vi "GrabImageDisplay.vi"(0 "nPixelFormat":i32, 1 "pInputBuffer":u8[](array[numeric]), 5 "nWidth":u32, 7 "nHeight":u32, 9 "Image Src":T1, 11 "error in (no error)":errorcluster) -> (4 "Image out":T1, 15 "error out":errorcluster)   [LabVIEW 2016, in "GxLVLib.lvlib"]
uses:
  GxLVLib.lvlib
  <vilib>/vision/Image Controls.llb/IMAQ Image.ctl
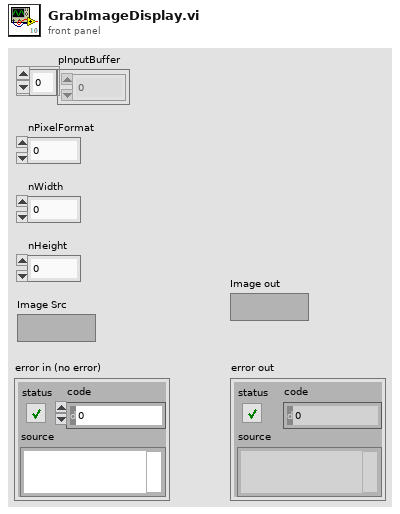
[diagram p1: front panel]
types:
  T1 = typedef "IMAQ Image.ctl" = refnum<image>
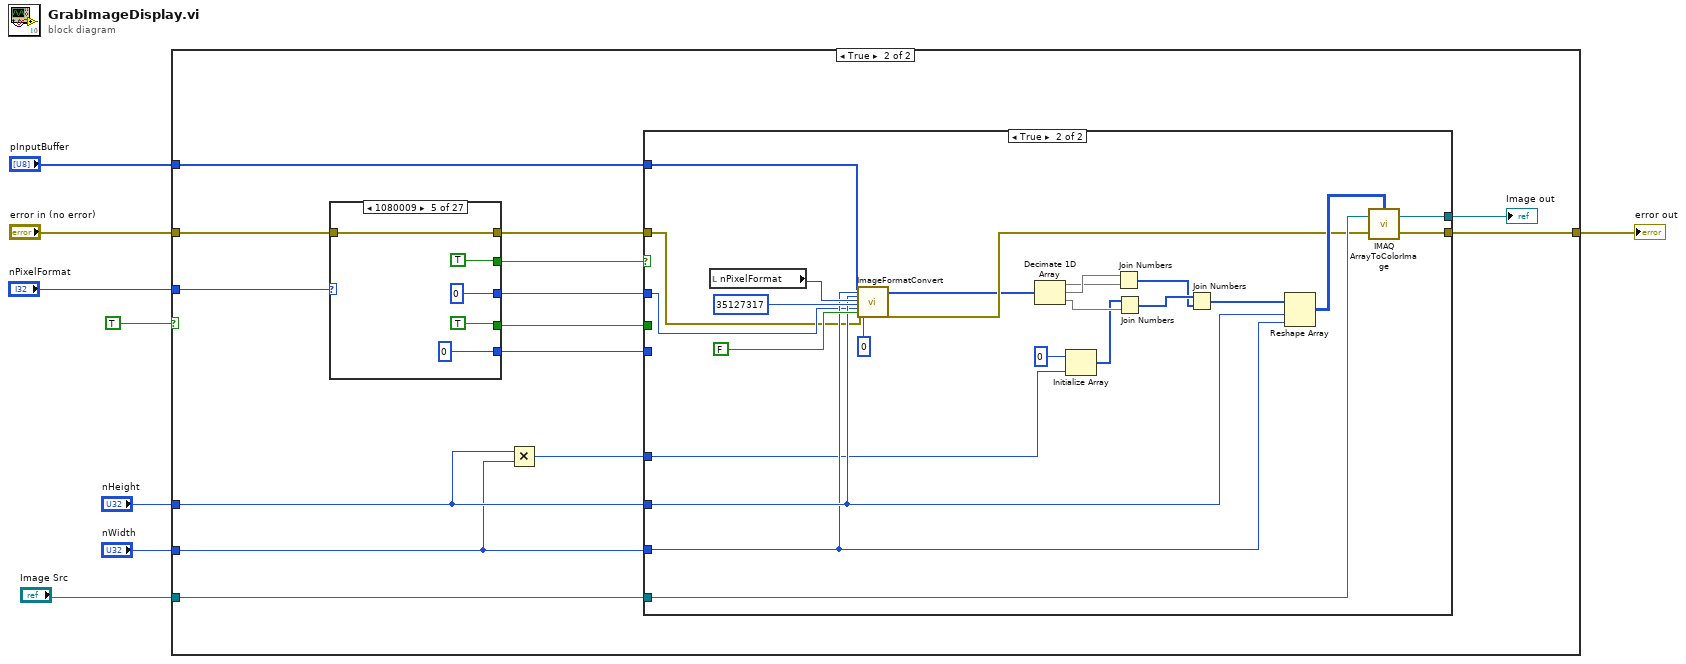
[diagram p0: block diagram]
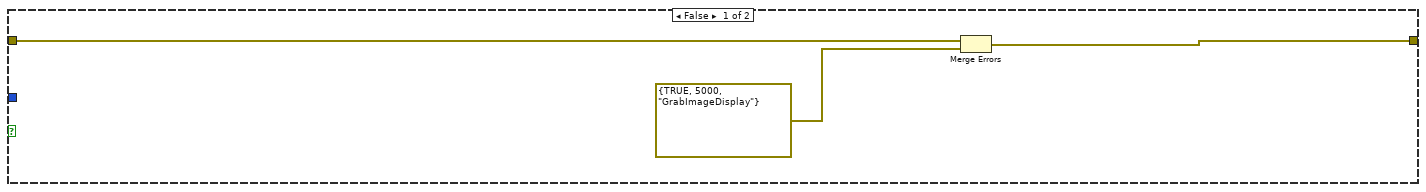
[diagram p2: hidden frame]
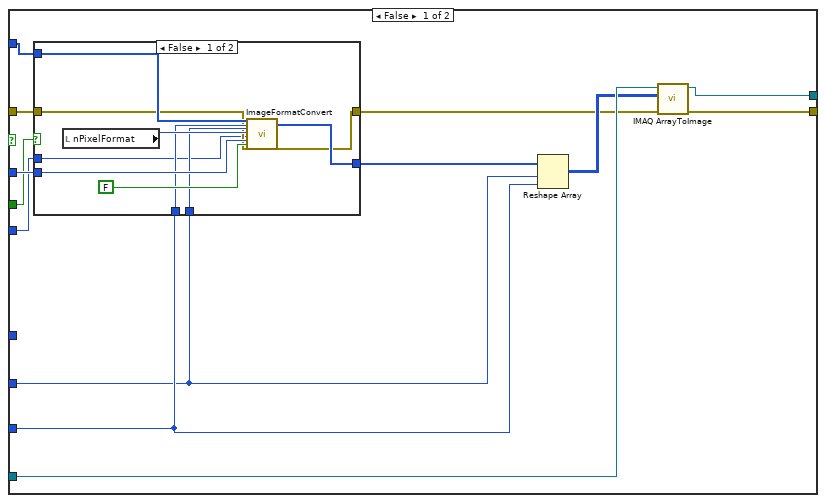
[diagram p3: hidden frame]
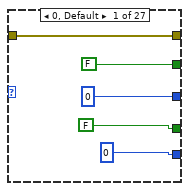
[diagram p5: hidden frame]
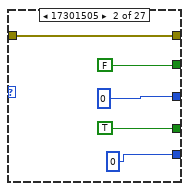
[diagram p6: hidden frame]
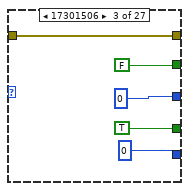
[diagram p7: hidden frame]
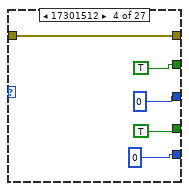
[diagram p8: hidden frame]
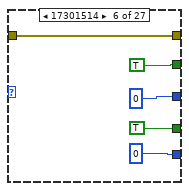
[diagram p9: hidden frame]
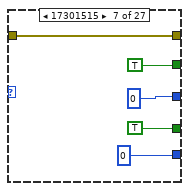
[diagram p10: hidden frame]
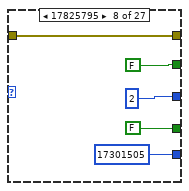
[diagram p11: hidden frame]
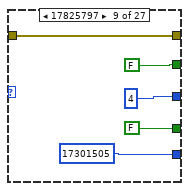
[diagram p12: hidden frame]
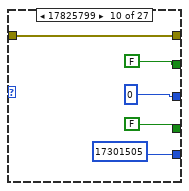
[diagram p13: hidden frame]
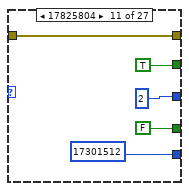
[diagram p14: hidden frame]
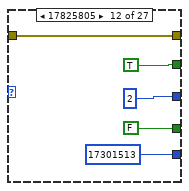
[diagram p15: hidden frame]
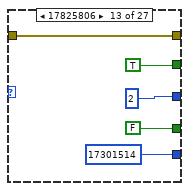
[diagram p16: hidden frame]
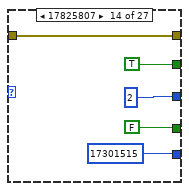
[diagram p17: hidden frame]
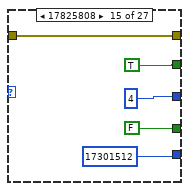
[diagram p18: hidden frame]
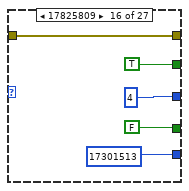
[diagram p19: hidden frame]
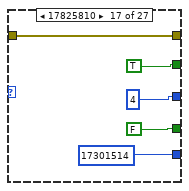
[diagram p20: hidden frame]
diagram:
  n1 = case shown="True" TRUE ("Boolean") {
    tunnel: "error in (no error)" -> [w11 w17]
    tunnel: [w9 w20] -> w7
    tunnel: "Image Src" -> [_ w21]
    tunnel: "nPixelFormat" -> [_ w16]
    tunnel: "nHeight" -> [_ w15]
    tunnel: "nWidth" -> [_ w14]
    tunnel: "pInputBuffer" -> [_ w13]
    frame False {
      n2 = Merge Errors(w11, errorcluster {TRUE, 5000, "GrabImageDisplay"}) -> (w9:errorcluster)
    }
    frame True {
      n3 = case shown="1080009" w16 {
        tunnel: [0 0 0 0 0 0 0 2 4 0 2 2 2 2 4 4 4 4 0 0 0 0 0 0 2 4 0] -> w24
        tunnel: [FALSE FALSE FALSE TRUE TRUE TRUE TRUE FALSE FALSE FALSE TRUE TRUE TRUE TRUE TRUE TRUE TRUE TRUE FALSE TRUE TRUE TRUE TRUE TRUE TRUE TRUE TRUE] -> w25
        tunnel: [FALSE TRUE TRUE TRUE TRUE TRUE TRUE FALSE FALSE FALSE FALSE FALSE FALSE FALSE FALSE FALSE FALSE FALSE FALSE FALSE FALSE FALSE FALSE FALSE FALSE FALSE FALSE] -> w23
        tunnel: w17 -> [w76 w81 w89 w94 w99 w104 w109 w114 w119 w124 w129 w134 w139 w144 w149 w154 w159 w164 w169 w174 w179 w184 w189 w194 w199 w204 w209]
        tunnel: [w76 w81 w89 w94 w99 w104 w109 w114 w119 w124 w129 w134 w139 w144 w149 w154 w159 w164 w169 w174 w179 w184 w189 w194 w199 w204 w209] -> w22
        tunnel: [0 ("DstPixelFormat") 0 ("DstPixelFormat") 0 ("DstPixelFormat") 0 ("DstPixelFormat") 0 ("DstPixelFormat") 0 ("DstPixelFormat") 0 ("DstPixelFormat") 17301505 ("DstPixelFormat") 17301505 ("DstPixelFormat") 17301505 ("DstPixelFormat") 17301512 ("DstPixelFormat") 17301513 ("DstPixelFormat") 17301514 ("DstPixelFormat") 17301515 ("DstPixelFormat") 17301512 ("DstPixelFormat") 17301513 ("DstPixelFormat") 17301514 ("DstPixelFormat") 17301515 ("DstPixelFormat") 17301505 ("DstPixelFormat") 17301512 ("DstPixelFormat") 17301513 ("DstPixelFormat") 17301514 ("DstPixelFormat") 17301515 ("DstPixelFormat") 0 ("DstPixelFormat") 0 ("DstPixelFormat") 0 ("DstPixelFormat") 0 ("DstPixelFormat")] -> w12
        frame 0, Default {
        }
        frame 17301505 {
        }
        frame 17301506 {
        }
        frame 17301512 {
        }
        frame 17301513 {
        }
        frame 17301514 {
        }
        frame 17301515 {
        }
        frame 17825795 {
        }
        frame 17825797 {
        }
        frame 17825799 {
        }
        frame 17825804 {
        }
        frame 17825805 {
        }
        frame 17825806 {
        }
        frame 17825807 {
        }
        frame 17825808 {
        }
        frame 17825809 {
        }
        frame 17825810 {
        }
        frame 17825811 {
        }
        frame 17825829 {
        }
        frame 17825838 {
        }
        frame 17825839 {
        }
        frame 17825840 {
        }
        frame 17825841 {
        }
        frame 35127329 {
        }
        frame 36700194 {
        }
        frame 36700195 {
        }
        frame 36700196 {
        }
      }
      n4 = Multiply(x=w15, y=w14) -> (x*y=w18:u32)
      n5 = case shown="True" w25 {
        tunnel: w24 -> [w38 w58]
        tunnel: w18 -> [_ w54]
        tunnel: w23 -> [w37 _]
        tunnel: w22 -> [w36 w57]
        tunnel: w21 -> [w35 w74]
        tunnel: [w33 w72] -> w20
        tunnel: [w32 w73] -> w19
        tunnel: w15 -> [w27 w60]
        tunnel: w14 -> [w28 w59]
        tunnel: w13 -> [w29 w55]
        tunnel: w12 -> [w26 _]
        frame False {
          n6 = case shown="False" w37 {
            tunnel: w38 -> [w46 _]
            tunnel: w36 -> [w41 w50]
            tunnel: [w40 w50] -> w31
            tunnel: [w47 w49] -> w30
            tunnel: w29 -> [w48 w49]
            tunnel: w28 -> [w43 _]
            tunnel: w27 -> [w42 _]
            tunnel: w26 -> [w39 _]
            frame False {
              n7 = local read "nPixelFormat"() -> (w44:i32)
              n8 = call "ImageFormatConvert.vi"("pInputBuffer"=w48, "nWidth"=w43, "nHeight"=w42, "nSrcPixelFormat"=w44, "nDstPixelFormat"=w39, "nValidBits"=w46, "bFlip"=FALSE ("Flip"), "error in (no error)"=w41) -> ("nOutputBuffer"=w47:u8[], "error out"=w40:errorcluster)  [unwired: 17 in, 1 out]
            }
            frame True {
            }
          }
          n9 = Reshape Array(w30, w27, w28) -> (w34:u8[][])
          n10 = call "IMAQ ArrayToImage"("error in (no error)"=w31, "Image Pixels (U8)"=w34, "Image"=w35) -> ("error out"=w33:errorcluster, "Image Out"=w32:T1)  [unwired: 7 in]
        }
        frame True {
          n11 = local read "nPixelFormat"() -> (w61:i32)
          n12 = call "ImageFormatConvert.vi"("pInputBuffer"=w55, "nWidth"=w59, "nHeight"=w60, "nSrcPixelFormat"=w61, "nDstPixelFormat"=35127317 ("DstPixelFormat"), "nValidBits"=w58, "bFlip"=FALSE, "error in (no error)"=w57, "nConvertType"=0 ("ConvertType")) -> ("nOutputBuffer"=w52:u8[], "error out"=w56:errorcluster)  [unwired: 16 in, 1 out]
          n13 = Decimate 1D Array(w52) -> (w68:u8[], w69:u8[], w67:u8[])
          n14 = Initialize Array(u8 0, w54) -> (w66:u8[])
          n15 = Join Numbers(hi=w69, lo=w68) -> ((hi.lo)=w64:u16[])
          n16 = Join Numbers(hi=w66, lo=w67) -> ((hi.lo)=w65:u16[])
          n17 = Join Numbers(hi=w65, lo=w64) -> ((hi.lo)=w51:u32[])
          n18 = Reshape Array(w51, w60, w59) -> (w71:u32[][])
          n19 = call "IMAQ ArrayToColorImage"("Image Pixels (U32)"=w71, "Image"=w74, "error in (no error)"=w56) -> ("Image Out"=w73:T1, "error out"=w72:errorcluster)  [unwired: 2 in]
        }
      }
      "Image out" <- w19
    }
  }
  "error out" <- w7
